vi "DAQmx Task Method.vi"() -> ()   [LabVIEW 2020]
uses:
  <vilib>/DAQmx/read.llb/DAQmx Read (Analog Wfm 1Chan NSamp).vi
  <vilib>/DAQmx/miscellaneous.llb/DAQmx Fill In Error Info.vi
panel:
  out "Data":waveform(dbl)(graph)
  in  "Number of Samples":i32=2560
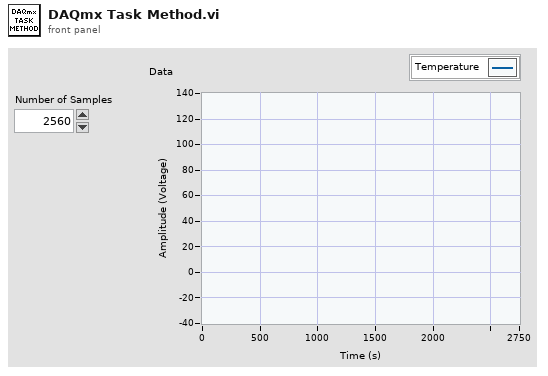
[diagram p1: front panel]
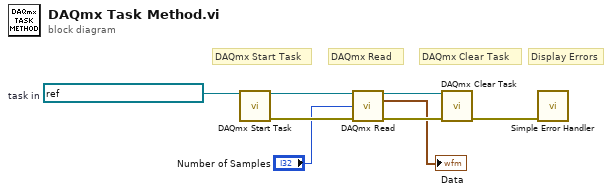
[diagram p0: block diagram]
diagram:
  w8 = refnum<k21> "My Analog Input Voltage"  # task in
  # "Display Errors"
  # "DAQmx Clear Task"
  # "DAQmx Read"
  # "DAQmx Start Task"
  n1 = call <vilib>:"DAQmx Start Task.vi"("task/channels in"=w8) -> ("task out"=w7:refnum<k21>, "error out"=w6:errorcluster)  [unwired: 13 in]
  n2 = call-poly <vilib>:"DAQmx Read.vi"("task/channels in"=w7, "number of samples per channel"="Number of Samples", "error in"=w6) -> ("task out"=w5:refnum<k21>, "data"=→"Data":waveform(dbl), "error out"=w4:errorcluster)  [unwired: 10 in]
  n3 = call <vilib>:"DAQmx Clear Task.vi"("task in"=w5, "error in"=w4) -> ("error out"=w1:errorcluster)  [unwired: 13 in]
  n4 = call <vilib>:"Simple Error Handler.vi"("error in (no error)"=w1) -> ()  [unwired: 4 in, 5 out]
